vi "Wait on Module Sync.vi"(8 "error in":errorcluster, 9 "Module ID":i32) -> (0 "error out":errorcluster)   [LabVIEW 2024, in "Camera.lvlib"]
doc: "Wait on the rendezvous that synchronizes the creation of the events.\n_____\nBased on DQMH Dev Tools: Project Template 7.1.0.1503."
uses:
  Camera.lvlib
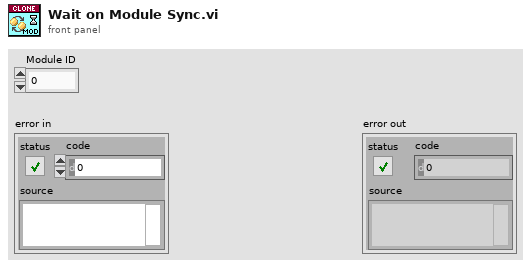
[diagram p1: front panel]
types:
  T1 = typedef "Rendezvous RefNum" = refnum<k1>
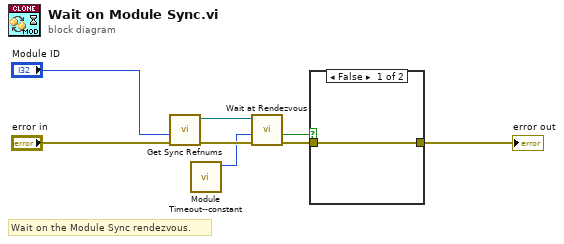
[diagram p0: block diagram]
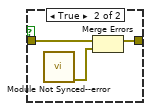
[diagram p2: hidden frame]
diagram:
  # "Wait on the Module Sync rendezvous."
  n1 = call "Get Sync Refnums.vi"("error in"="error in", "Module ID"="Module ID") -> ("error out"=w6:errorcluster, "Module Sync"=w7:T1)  [unwired: 6 in, 2 out]
  n2 = call "Module Timeout--constant.vi"() -> ("Module Timeout"=w5:i32)  [unwired: 11 in]
  n3 = call <vilib>:"Wait at Rendezvous.vi"("error in (no error)"=w6, "ms timeout (-1)"=w5, "rendezvous"=w7) -> ("error out"=w3:errorcluster, "timed out"=w2:bool)  [unwired: 2 in, 1 out]
  n4 = case shown="False" w2 {
    tunnel: w3 -> [w9 w12]
    tunnel: [w9 w11] -> w1
    frame False {
    }
    frame True {
      n5 = call "Module Not Synced--error.vi"() -> ("error out"=w10:errorcluster)  [unwired: 11 in]
      n6 = Merge Errors(w12, w10) -> (w11:errorcluster)
    }
  }
  "error out" <- w1
